vi "PwF_ToF_GetCalState.vi"(0 "PwF ToF Ref":T1, 11 "error in (no error)":errorcluster) -> (4 "PwF ToF Ref":T1, 6 "OpticalCenter_X":u8, 8 "OpticalCenter_Y":u8, 10 "RangeOffset_mm":u16, 15 "error out":errorcluster)   [LabVIEW 2018]
uses:
  ToF_TypeDef/PwF ToF Ref.ctl
  ToF_TypeDef/PwF ToF RangingMode.ctl
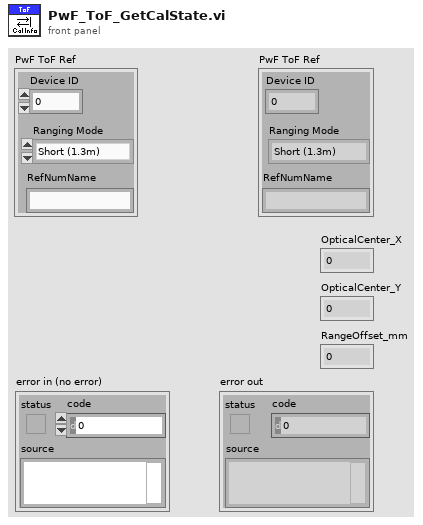
[diagram p1: front panel]
types:
  T1 = typedef "PwF ToF Ref.ctl" = cluster{"Device ID":u8, "Ranging Mode":T2, "RefNumName":string}
  T2 = typedef "PwF ToF RangingMode.ctl" = enum8{"Short (1.3m)", "Medium (2m)", "Long (4m)"}
  T3 = cluster{"Data[0]":u8, "Data[1]":u8, "Data[2]":u8, "Data[3]":u8, "Data[4]":u8, "Data[5]":u8, "Data[6]":u8, "Data[7]":u8, "Data[8]":u8}
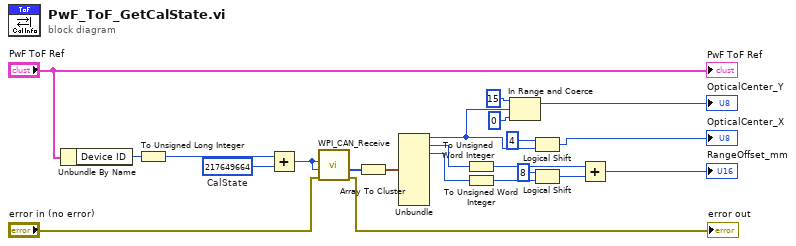
[diagram p0: block diagram]
diagram:
  w20 = u32 217649664  # CalState
  n1 = Unbundle By Name("PwF ToF Ref") -> ("Device ID"=w22:u8)
  n2 = To Unsigned Long Integer(number=w22) -> (unsigned 32bit integer=w1:u32)
  n3 = Add(x=w1, y=w20) -> (x+y=w19:u32)
  n4 = call <vilib>:"WPI_CAN_Receive.vi"("error in (no error)"="error in (no error)", "Message ID Mask"=w19, "Message ID"=w19) -> ("error out"=→"error out":errorcluster, "Data"=w17:u8[])  [unwired: 6 in, 1 out]
  n5 = Array To Cluster(array=w17) -> (cluster=w18:T3)
  n6 = Unbundle(w18) -> ("Data[0]"=w4:u8, "Data[1]"=w12:u8, "Data[2]"=w11:u8)  [unwired: 6 out]
  n7 = To Unsigned Word Integer(number=w12) -> (unsigned 16bit integer=w13:u16)
  n8 = To Unsigned Word Integer(number=w11) -> (unsigned 16bit integer=w10:u16)
  n9 = In Range and Coerce(upper limit=u8 15, x=w4, lower limit=u8 0) -> (coerced(x)=→"OpticalCenter_Y":u8)  [unwired: 1 out]
  n10 = Logical Shift(y=i16 4, x=w4) -> (x << y=→"OpticalCenter_X":u8)
  n11 = Logical Shift(y=i16 8, x=w10) -> (x << y=w15:u16)
  n12 = Add(x=w13, y=w15) -> (x+y=→"RangeOffset_mm":u16)
  "PwF ToF Ref" <- "PwF ToF Ref"
